vi "Periodic Tasks.vi"   [LabVIEW 2017]
doc: "This VI runs in parallel to other tasks. It can contain as many user-defined periodic loops as you need. These can carry out PID or other sorts of timed response."
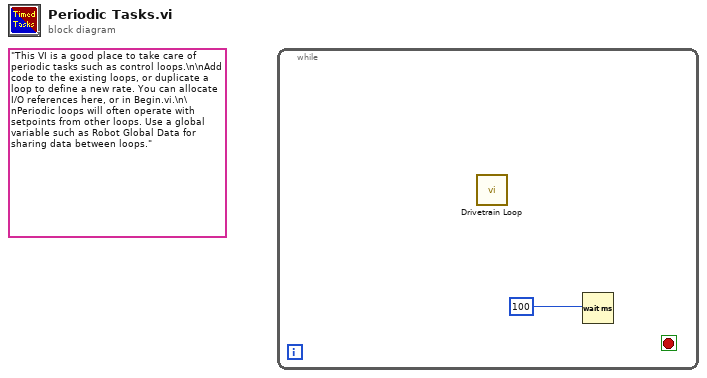
[diagram p0: block diagram]
diagram:
  (unwired) "This VI is a good place to take care of periodic tasks such as control loops.\n\nAdd code to the existing loops, or duplicate a loop to define a new rate. You can allocate I/O references here, or in Begin.vi.\n\nPeriodic loops will often operate with setpoints from other loops. Use a global variable such as Robot Global Data for sharing data between loops."
  n1 = while {
    stop <- _ stop-if-true
    n2 = call "Drivetrain Loop.vi"() -> ()  [unwired: 12 in]
    n3 = Wait (ms)(milliseconds to wait=100) -> ()  [unwired: 1 out]
  }
